vi "Process Data In Pipeline.vi"(8 "error in (no error)":errorcluster, 10 "AbstractData in":refnum<class "AbstractData.lvclass">, 11 "Pipelined Actor in":refnum<class "Pipelined Actor.lvclass">) -> (0 "error out":errorcluster, 2 "AbstractData out":refnum<class "AbstractData.lvclass">, 3 "Pipelined Actor out":refnum<class "Pipelined Actor.lvclass">)   [LabVIEW 2013, in "Pipelined Actor.lvlib" / "Pipelined Actor.lvclass"]
uses:
  Pipelined Actor.lvclass
  Data/Data Abstraction Layer/AbstractData/AbstractData.lvclass
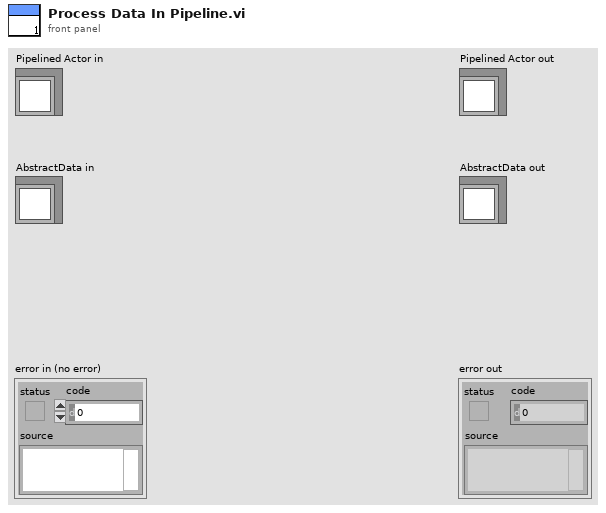
[diagram p1: front panel]
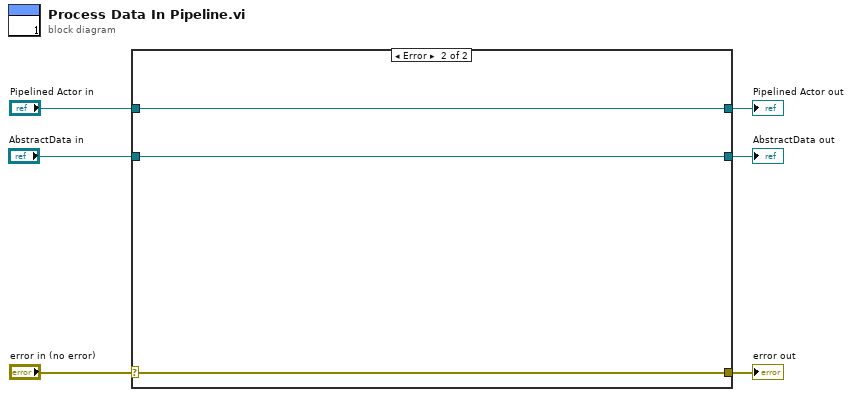
[diagram p0: block diagram]
diagram:
  n1 = case shown="Error" "error in (no error)" {
    selector: "error in (no error)" -> [w8 w12]
    tunnel: [w8 w12] -> w5
    tunnel: [w9 w11] -> w3
    tunnel: "Pipelined Actor in" -> [w9 w11]
    tunnel: "AbstractData in" -> [w7 w10]
    tunnel: [w7 w10] -> w1
    frame No Error {
      # "Wire the error cluster across even in the \"No Error\"\ncase so that warnings get propagated."
    }
    frame Error {
    }
  }
  "error out" <- w5
  "Pipelined Actor out" <- w3
  "AbstractData out" <- w1
